vi "laplacian.vi"(9 "zshape":i32[](array[numeric]), 10 "xshape":i32[](array[numeric]), 11 "input":sgl[](array[numeric])) -> (3 "output":sgl[](array[numeric]))   [LabVIEW 2013]
uses:
  imagereconstruction/x64/Debug/labviewdll.dll
panel:
  out "error":i32
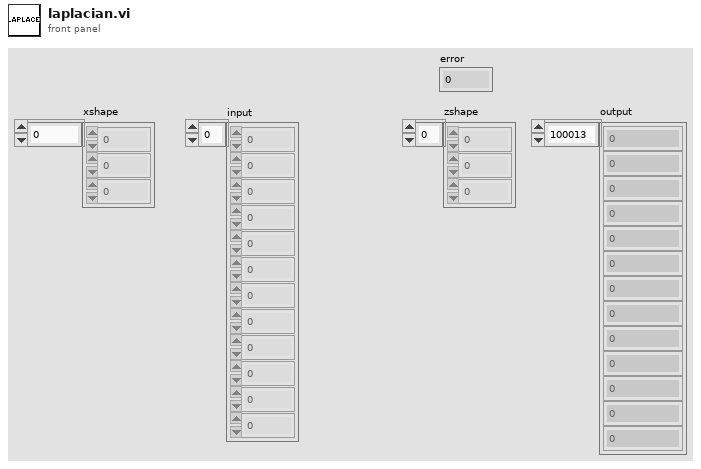
[diagram p1: front panel]
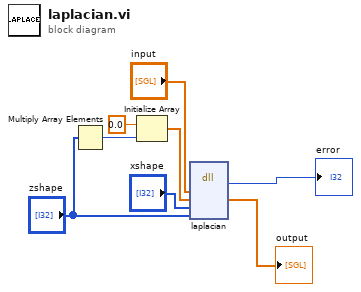
[diagram p0: block diagram]
diagram:
  n1 = Multiply Array Elements(1:"zshape") -> (0:w4:i32)
  n2 = Initialize Array(sgl 0.0 ("element"), w4) -> (w2:sgl[])
  n3 = dll-call lib="D:/work/uni/FYP/reconrepo/imagereconstruction/x64/Debug/labviewdll.dll" fn="laplacian"("input"="input", "output"=w2, "xshape"="xshape", "zshape"="zshape") -> ("return type"=→"error":i32, "output"=→"output":sgl[])  [unwired: 6 in, 2 out]
